vi "AlliGator Phasor Graph Context Menu Handler.vi"(8 "Error In":errorcluster, 9 "Help?":bool, 10 "Dialog? (T)":bool=TRUE, 11 "XY Graph Event":T3) -> (0 "Error Out":errorcluster, 1 "Message":string, 3 "AlliGator Actions":T1[](array[typedef]))   [LabVIEW 2021, in "AlliGator Phasor Graph.lvlib"]
doc: "Interprets Phasor Graph right-clic k menu items and sends corresponding actions to the action queue."
uses:
  AlliGator Phasor Graph.lvlib
  Graphs/XY Graph/XY Graph Event.ctl
  <vilib>/Utility/miscctls.llb/LVPoint32TypeDef.ctl
  AlliGator Q Element.ctl
  AlliGator Q Event.ctl
  Graphs/XY Graph/New Plot Information.ctl
  Graphs/Plot Scales.ctl
  Graphs/LabVIEW Plot Interpolation.ctl
  Graphs/Plot Point Style.ctl
  Graphs/XY Graph/XY Graph Selected Plot Info.ctl
  Graphs/XY Graph/XY Graph Refnum.ctl
  Graphs/XY Graph/XY Graph Mouse Click Event Data.ctl
  AlliGator Phasor Reference Data.ctl
  AlliGator Phasor Plot Scatter Plot Parameters.ctl
  AlliGator Phasor Graph Parameter List.ctl
  AlliGator Action Engine.lvlib
  Graphs/XY Graph/XY Graph Add-Ons.lvlib
  AlliGator Phasor Ratio.lvlib
  AlliGator Python Plugins.lvlib
  Graphs/Graphs.lvlib
panel:
  # "see the AlliGator License on the block diagram (Ctrl+E or Window:Show Block Diagram)"
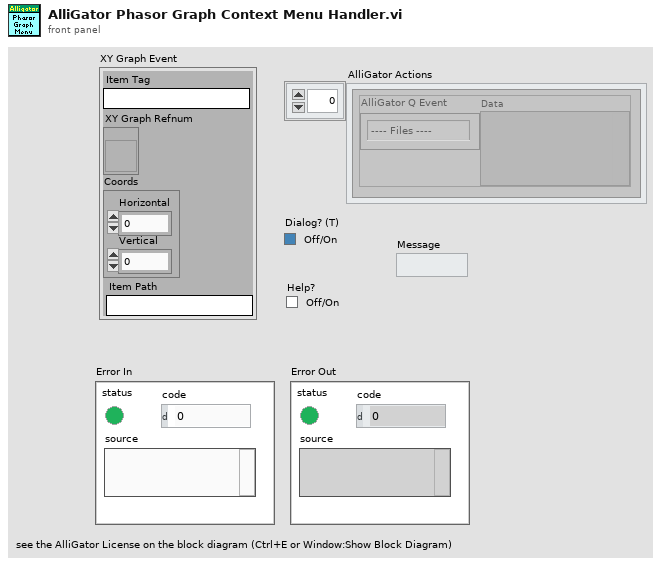
[diagram p1: front panel]
types:
  T1 = typedef "AlliGator Action Engine.lvlib/AlliGator Q Element.ctl" = cluster{"AlliGator Q Event":T2, "Data":variant}
  T2 = typedef "AlliGator Action Engine.lvlib/AlliGator Q Event.ctl" = enum16{"---- Files ----", "Files:Set Batch Export Files To Save", "Files:Set Dataset Loading & Pre-processing Options", "Files:Check #Frames in Dataset", "Files:Increment Frame Index", "Files:Open Mask Image", "Files:Open White Light Image", "Files:Open Single Dataset", "Files:New Folder of Folders Selected", "Files:Load File (all Types)_Scriptable", "Files:Move Flattened Series to Folders Series", "Files:Select Folder", "Files:Load FLI Dataset", "Files:Load Swiss SPAD 1 Dataset", "Files:Load Swiss SPAD 2 Dataset", "Files:Load .sdt FLI Dataset", "Files:Load .ptu FLI Dataset", "Files:Load .bin FLI Dataset", "Files:Load Single Gate Image Folder", "Files:Load I/m/phi Dataset (deprecated)", "Files:Load Single Image", "Files:Subtract Background File", "Files:Export FLI Dataset", "Files:Load HDF5 FLI Dataset", "Files:Set Destination File Path", "Files:Save Mask Image", "Files:Batch Conversion", "Files:New Folder Selected", "Files:Close FLI Dataset", "Files:Close FLI Dataset Series", "Files:Close White Light Image", "Files:Close Mask Image", "---- FLI Dataset ----", "FLI Dataset:Channel Arithmetic", "FLI Dataset:Export Average Lifetime Map as ASCII", "FLI Dataset:Export User-Defined Quantity Map as ASCII", "FLI Dataset:Python Function FLI Dataset Event", "FLI Dataset:ROI Analysis", "FLI Dataset:Tilted Logistic Square Gated IRF Characteristics Map", "FLI Dataset:Logistic Square Gated IRF Characteristics Map", "FLI Dataset:Square Gated IRF Characteristics Map", "FLI Dataset:Multi-ROI Single-Pixel Phasor Analysis", "FLI Dataset:Multi-ROI Single-Pixel NLSF Analysis", "FLI Dataset:All ROIs IRF Extraction", "FLI Dataset:All ROIs Decay Fit Non-Interactive (Fast + Individual IRF)", "FLI Dataset:All ROIs Phasor Analysis", "FLI Dataset:All ROIs Decay Fit", "FLI Dataset:Fluorescence Decay Statistics", "FLI Dataset:Update Decay Statistics Graph", "FLI Dataset:Get Decay from ROI", "FLI Dataset:All ROIs Average Lifetimes", "---- FLI Dataset Series ----", "FLI Dataset Series:Sum All Datasets in Series", "FLI Dataset Series:Add Dataset to Accumulated Dataset", "FLI Dataset Series:Display Accumulated Dataset", "FLI Dataset Series:Clear Dataset Series Sum", "FLI Dataset Series:Time-Series Analysis (NLSF)", "FLI Dataset Series:Time-Series Analysis (Phasor)", "---- Image ----", "Image:Update Image Profile Plots", "Image:Image Histogram Cursor Move", "Image:Image Histogram", "Image:Image Contrast", "Image:Set Image Histogram Cursor Move Flag", "Image:Clear Image Overlay", "Image:Use ROI as Search Area", "Image:Set ROI Diameter", "Image:Save Image Data as TIFF", "Image:Save Displayed Image with Overlay", "Image:Save Image Overlay Only", "Image:Save Image as Hot Pixel Mask", "Image:Change Source Image Color Palette", "Image:Copy Image to Clipboard", "Image:Source Image ROI Selection", "Image:Delete All ROIs", "Image:Delete All Unselected ROIs", "Image:Delete ROI", "Image:Merge All ROIs", "Image:Store ROI", "Image:Source Image ROI Storage", "Image:Export ROI Description to Notebook", "Image:Save ROI", "Image:Load ROI", "Image:Paste ROI Definition", "Image:Clear ROI", "Image:Identify ROIs in Mask Image", "Image:Create Complementary ROI", "Image:Create Contour ROI", "Image:Create ROI(s) from Pixels with Peak above Min_Scriptable", "Image:Create ROI(s) from Pixels with Intensity above Min_Scriptable", "Image:Compute ROI Statistics", "Image:Delete ROI(s) based on ROI Characteristics", "Image:Create ROI Grid", "Image:ROI to Individual Pixel ROIs", "Image:Python Function Source Image Event", "Image:Show Phasor Calibration Map ROI Centers", "Image:Convert ROI to Mask Image", "Image:Mouse Move", "Image:Mouse Up", "Image:Set Source Image Mouse Move Flag", "Image:Add Scale Bar Overlay", "Image:Delete Existing ROIs Option", "---- Decay ----", "Decay:Clear IRF/Reference Plot", "Decay:Clear Local IRFs", "Decay:Add Decay to Graph", "Decay:Smoothen Plot", "Decay:Smoothen Plot Tail", "Decay:Average Selected Plots", "Decay:Extract IRF", "Decay:Optimal IRF Extraction", "Decay:Threshold IRF", "Decay:Fit to Model IRF", "Decay:Fit IRF to Square Gate", "Decay:Fit IRF to Logistic Square Gate", "Decay:Fit IRF to Tilted Logistic Square Gate", "Decay:Create Bounding Cursors Set", "Decay:Export Bounding Cursors Definition to Notebook", "Decay:Denoise Plot", "Decay:Compute Cumulative Function", "Decay:Use as Reference Decay", "Decay:Show Reference Decay/IRF", "Decay:Extrapolate Decay", "Decay:Create Head & Tail Bounding Cursors", "Decay:Store Cursor-defined Head & Tail Fractions", "Decay:Rebin Plot", "Decay:1-Normalize Decay", "Decay:[0-1]-Normalize Plot", "Decay:Straighten Decay", "Decay:Shift Decay", "Decay:Fold Decay", "Decay:Fit Decay", "Decay:Global Fit of Selected Decays", "Decay:Post Global Fit Script", "Decay:Add Global Fit Parameters to Graph", "Decay:Add Decay Parameter(s) to Plot (Graph)", "Decay:Export Decay to Phasor Graph", "Decay:Plot Decay Shifts", "Decay:Compute Average Lifetime", "Decay:Plot Convolution", "Decay:Graph Tip Strip Update", "---- Decay Statistics ----", "Decay Statistics:Tip Strip Update", "---- Intensity Time Trace ----", "Intensity Time Trace:Use File Timestamp", "Intensity Time Trace:Load Intensity Corrections File", "Intensity Time Trace:Clear Intensity Corrections File", "Intensity Time Trace:Tip Strip Update", "---- Phasor Plot ----", "Phasor Plot:Build Phasor Plot", "Phasor Plot:Change Phasor Plot Color Palette", "Phasor Plot:Adjust Phasor Plot Display Range", "Phasor Plot:Highlight Image ROI in Phasor Plot", "Phasor Plot:Save Phasor Plot Image with Overlay", "Phasor Plot:Export Complex Phasor Map", "Phasor Plot:Export Phasor Ratio Map", "Phasor Plot:Export Average Lifetime Map", "Phasor Plot:Compute Phase Lifetime Histogram", "Phasor Plot:Compute Phasor Ratio Histogram", "Phasor Plot:Compute Phase Lifetime vs Intensity Scatter Plot", "Phasor Plot:Weber 2-Component Decomposition", "Phasor Plot:Update Phasor Color Map Vertices", "Phasor Plot:Clear Phasor Overlay", "Phasor Plot:Use Segment Extremities as References", "Phasor Plot:Use UC/Segment Intersections as References", "Phasor Plot:Use UC/Principal Axis Intersections as References", "Phasor Plot:Use UC/Linear Fit Intersections as References", "Phasor Plot:Update Phasor Plot Reference", "Phasor Plot:Show Local Phasor Info in Phasor Plot", "Phasor Plot:Update Phasor Plot State", "Phasor Plot:Phasor Plot ROI Storage", "Phasor Plot:Phasor Plot ROI Selection", "Phasor Plot:Python Function Phasor Plot Event", "Phasor Plot:Overlay Phasor ROI, Ratio or Map in Source Image", "Phasor Plot:Phasor at Image Pixel", "Phasor Plot:Mouse Move", "Phasor Plot:Mouse Up", "Phasor Plot:Display Range Mouse Move", "Phasor Plot:Set Mouse Move Flag", "---- Phasor Graph ----", "Phasor Graph:Calibrated Phasor Map Series", "Phasor Graph:Whole Image Phasor Scatter Plot (Todo)", "Phasor Graph:Get Phasor Value", "Phasor Graph:Create New Phasor Plot Dialog", "Phasor Graph:Update Last Phasor Value", "Phasor Graph:Update Phasor (m, phi)", "Phasor Graph:Remove Single Phasor from Plot", "Phasor Graph:Add Single Phasor to Plot", "Phasor Graph:Remove Phasor Plot", "Phasor Graph:Remove Selected Phasor Plots", "Phasor Graph:Clear Phasor Data", "Phasor Graph:Clear Phasor Graph", "Phasor Graph:Cursor Move", "Phasor Graph:Draw Cursor Connecting Line", "Phasor Graph:Clear Cursor Connecting Line", "Phasor Graph:Find UC Intersection", "Phasor Graph:Use UC/Cursor-Defined Line Intersections", "Phasor Graph:Use Selected Plots Fitted Line/UC Intersections", "Phasor Graph:Use Selected Plots Principal Axis/UC Intersections", "Phasor Graph:Show Single Phasor", "Phasor Graph:Save Single Phasor Plot", "Phasor Graph:Save All Phasor Plots", "Phasor Graph:Load Phasor Plot(s)", "Phasor Graph:Phasor Multiplication", "Phasor Graph:Compute Average Phasor", "Phasor Graph:Compute Multiple Average Phasors (Selected Plots)", "Phasor Graph:Export Single Phasor Plot Phase Lifetimes", "Phasor Graph:Phase Lifetime Trajectory", "Phasor Graph:Phase Lifetime vs Intensity Scatter Plot (deprecated)", "Phasor Graph:Parameter 2 vs Parameter 1 Scatter Plot", "Phasor Graph:Use Cursor n Location", "Phasor Graph:Set Reference n to Current Phase Lifetime Value", "Phasor Graph:Set Reference n to Lifetime Value", "Phasor Graph:Set Cursor n Location", "Phasor Graph:Save Phasor Graph Image", "Phasor Graph:Update SEPL Plot", "Phasor Graph:Export Single Phasor Plot Data", "Phasor Graph:Export Selected Phasor Plots Data", "Phasor Graph:Python Function Phasor Graph Event", "Phasor Graph:Tip Strip Update", "---- Calibration ----", "Calibration:Set Calibration Type", "Calibration:Load/Save Phasor Calibration", "Calibration:Load/Save Phasor Calibration Series", "Calibration:Load/Save Phasor Calibration Map", "Calibration:Use as Calibration", "Calibration:Compute Optimal Calibration from Phasor References", "Calibration:Clear Phasor Calibration", "Calibration:Use as Calibration Series", "Calibration:Use as Calibration Map", "Calibration:Clear Calibration Series", "Calibration:Clear Calibration Map", "Calibration:Apply Phasor Calibration", "Calibration:Update Single Plot Calibration", "Calibration:Update Multiple Plots Calibration", "Calibration:Clear Single Plot Calibration", "Calibration:Clear All Plots Calibrations", "Calibration:Clear Plot(s) Calibration(s)?", "Calibration:Phasor Calibration Maps (# Gates Series)", "---- Phasor Ratio ----", "Phasor Ratio:Clear Reference n", "Phasor Ratio:Toggle Selected Plot(s)  Lock to Reference 1", "Phasor Ratio:Use as Reference n", "Phasor Ratio:Send Reference n to Notebook", "Phasor Ratio:Toggle Selected Plot(s)  Lock to Reference 2", "Phasor Ratio:Compute Phasor Ratio at Mouse Location", "Phasor Ratio:Compute Phasor Plot's Average Phasor Ratio", "Phasor Ratio:Compute Time-Series Phasor Ratios", "Phasor Ratio:Fit Line to Phasor Ratio Plot", "Phasor Ratio:Save References", "Phasor Ratio:Load References", "Phasor Ratio:Update Phasor Reference 1", "Phasor Ratio:Update Phasor Reference 2", "Phasor Ratio:Move Cursor n to Reference n", "Phasor Ratio:Use as Phasor Reference 1 Lifetime", "Phasor Ratio:Use as Phasor Reference 2 Lifetime", "Phasor Ratio:Export Phasor Ratio Map as ASCII", "Phasor Ratio:Tip Strip Update", "---- Lifetime & Other Parameters Graph ----", "Lifetime:Tip Strip Update", "---- Decay Fit Parameter Map ----", "Decay Fit Parameter Map:Export ROI NLSF Data as ASCII", "Decay Fit Parameter Map:Set Decay Fit  Parameter Map Selection", "Decay Fit Parameter Map:Build Decay Fit Parameter Map", "Decay Fit Parameter Map:Change Decay Fit Parameter Map Color Palette", "Decay Fit Parameter Map:Export Decay Fit Parameter Map Data as ASCII", "Decay Fit Parameter Map:Export All Decay Fit Parameter Maps Data as ASCII", "Decay Fit Parameter Map:Send Map Data to Lifetime Graph", "Decay Fit Parameter Map:Save Decay Fit Parameter Map Image", "Decay Fit Parameter Map:Save-Load IRFs & Fit Data", "Decay Fit Parameter Map:Update Local Decay Plots", "Decay Fit Parameter Map:Python Function Decay Fit Parameters Map Event", "Decay Fit Parameter Map:Overlay Decay Fit Parameter Map in Source Image", "Decay Fit Parameter Map:Plot Map Data vs Intensity", "Decay Fit Parameter Map:Mouse Up", "Decay Fit Parameter Map:Display Range Mouse Move", "---- Generic Graph ----", "Generic Graph:Generic XY Graph Event", "Generic Graph:Python Function XY Graph Event", "Generic Graph:New Plot", "Generic Graph:Save Plot", "Generic Graph:XY Plot Histogram", "Generic Graph:Set XY Graph Plot Name", "Generic Graph:Set Last Cursor Style", "Generic Graph:Tip Strip Update", "---- GUI ----", "GUI:Start Script", "GUI:Type of Displayed Image Changed", "GUI:Gate Image Slide Changed", "GUI:Show Busy Icon", "GUI:Show Busy Icon & Abort Button", "GUI:Hide Busy Icon", "GUI:Hide Busy Icon & Abort Button", "GUI:Abort", "GUI:End Script", "GUI:Start Timing", "GUI:End Timing", "GUI:Set State Indicator", "GUI:Send Parameters JSON Strings to Clipboard", "GUI:Set Gate Step", "GUI:Idle", "GUI:Initialization", "GUI:Quit", "GUI:Increment Dataset Index", "GUI:Set Dataset Index to -1", "GUI:Time Series Slider Moved", "GUI:Time Series Slider Changed", "GUI:Toggle Playback or Loop", "GUI:Playback Script", "GUI:Set Phasor Frequency", "GUI:Open Window", "DEBUG"}
  T3 = typedef "XY Graph Add-Ons.lvlib/XY Graph Event.ctl" = cluster{"Item Tag":string, "XY Graph Refnum":refnum<vi>, "Coords":T4, "Item Path":string}
  T4 = typedef "LVPoint32TypeDef.ctl" = cluster{"Horizontal":i32, "Vertical":i32}
  T5 = typedef "XY Graph Add-Ons.lvlib/New Plot Information.ctl" = cluster{"Multiplot XY Graph":refnum<vi>, "Plot Name":string, "Plot Scales":T6, "Plot Interpolation":T7, "Point Style":T8, "Plot Color":u32, "Plot Metadata":variant}
  T6 = typedef "XY Graph Add-Ons.lvlib/Plot Scales.ctl" = cluster{"X Scale":u32, "Y Scale":u32}
  T7 = typedef "Graphs.lvlib/LabVIEW Plot Interpolation.ctl" = u8
  T8 = typedef "Graphs.lvlib/Plot Point Style.ctl" = enum16{"not defined", "None", "Empty Circle", "Filled Circle", "Thick Circle", "Dotted Circle", "Empty Square", "Filled Square", "Thick Square", "Dotted Square", "Small Filled Square", "Dot", "Cross", "Tiny Cross", "Large X", "Small x", "Diamond", "Small Empty Square"}
  T9 = typedef "XY Graph Add-Ons.lvlib/XY Graph Selected Plot Info.ctl" = cluster{"Multiplot XY Graph":T10, "Mouse Coordinates":T4, "Plot Index":i32}
  T10 = typedef "XY Graph Add-Ons.lvlib/XY Graph Refnum.ctl" = refnum<vi>
  T11 = typedef "XY Graph Add-Ons.lvlib/XY Graph Mouse Click Event Data.ctl" = cluster{"Multiplot XY Graph":T10, "Mouse Coordinates":T4}
  T12 = typedef "AlliGator Phasor Ratio.lvlib/AlliGator Phasor Reference Data.ctl" = cluster{"Data Type":string, "Data":variant}
  T13 = cluster{"Mouse Click Event Data":T11, "Save as...":bool}
  T14 = cluster{"XY Graph Refnum":refnum<vi>, "Coords":T4}
  T15 = cluster{cluster{"XY Graph Refnum":refnum<vi>, "Coords":T4}, i32}
  T16 = typedef "AlliGator Phasor Graph.lvlib/AlliGator Phasor Plot Scatter Plot Parameters.ctl" = cluster{"Parameter 2":T17, "Parameter 1":T17}
  T17 = typedef "AlliGator Phasor Graph.lvlib/AlliGator Phasor Graph Parameter List.ctl" = enum16{"Time Stamp", "Index", "Phasor Parameters", "Phasor g", "Phasor s", "Phasor phi", "Phasor m", "Modulus Lifetime", "Phase Lifetime", "ROI Parameters", "ROI Center x", "ROI Center y", "ROI # pixels ", "Decay Parameters", "Intensity", "Background/Gate", "Intensity - Background", "Fitted Lifetime", "Fitted Intensity", "Phasor Ratio Parameters", "Amplitude Phasor Ratio", "Intensity Phasor Ratio", "Amplitude-Averaged Lifetime", "Intensity-Averaged Lifetime", "-", "Phasor Parameters SDV", "Phasor g SDV", "Phasor s SDV", "Phasor phi SDV", "Phasor m SDV", "Phase Lifetime SDV", "Modulus Lifetime SDV", "Phasor Ratio Parameters SDV", "Amplitude Phasor Ratio SDV", "Intensity Phasor Ratio SDV", "Amplitude-Averaged Lifetime SDV", "Intensity-Averaged Lifetime SDV"}
  T18 = cluster{"Selected Plot Info":T9, "Dummy Scatter Plot Parameters\nindicating that a Dialog":T16}
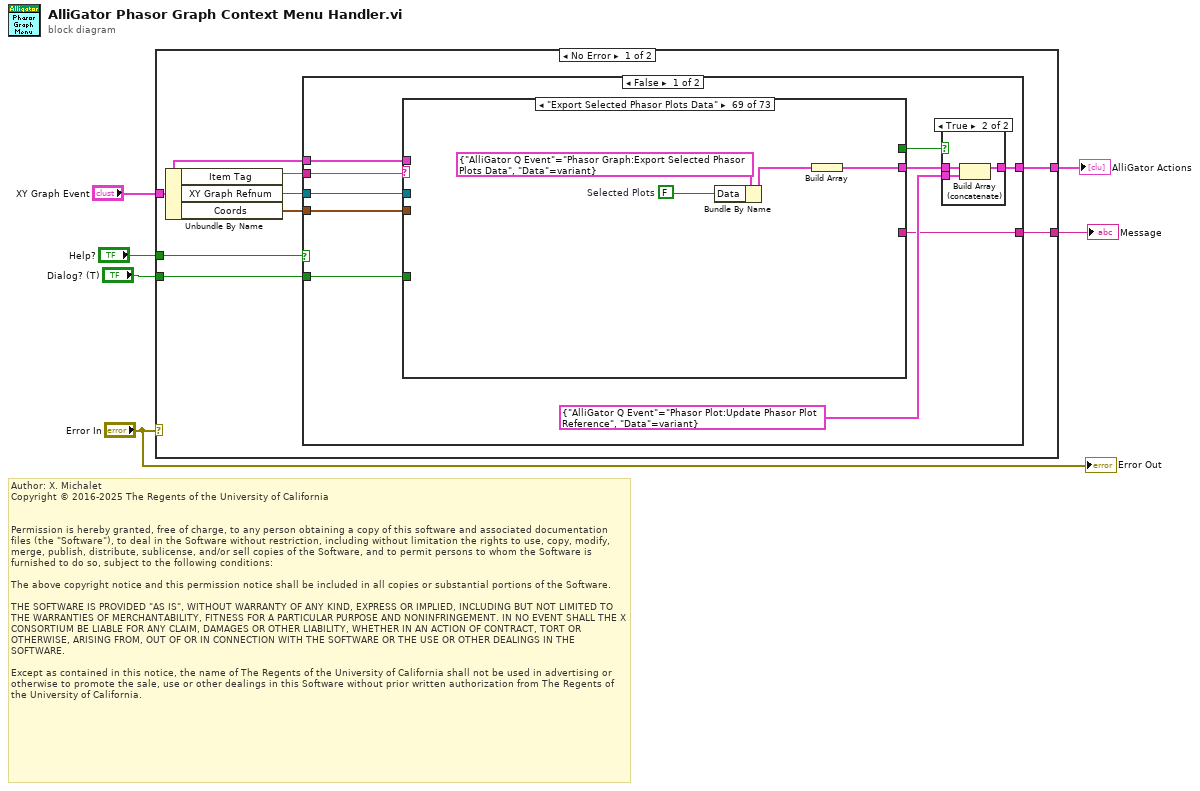
[diagram p0: block diagram]
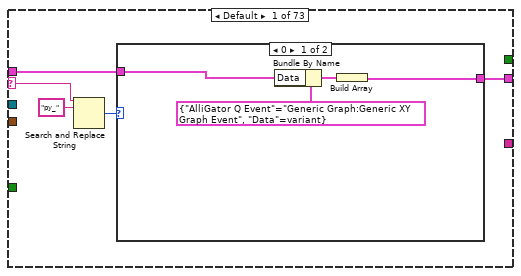
[diagram p3: hidden frame]
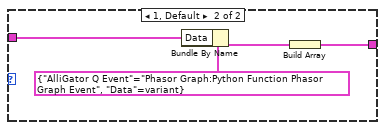
[diagram p4: hidden frame]
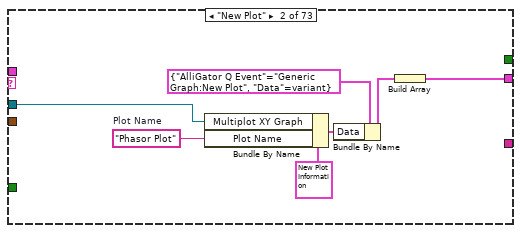
[diagram p5: hidden frame]
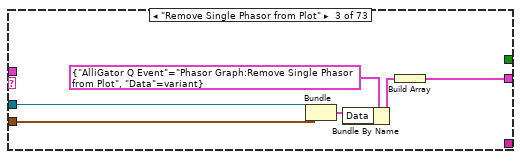
[diagram p6: hidden frame]
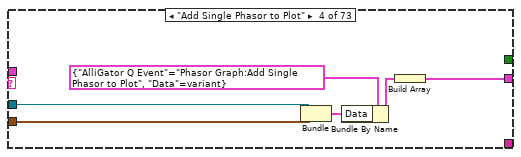
[diagram p7: hidden frame]
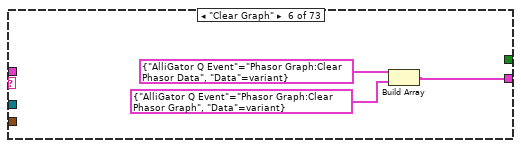
[diagram p9: hidden frame]
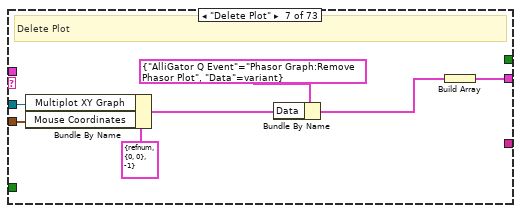
[diagram p10: hidden frame]
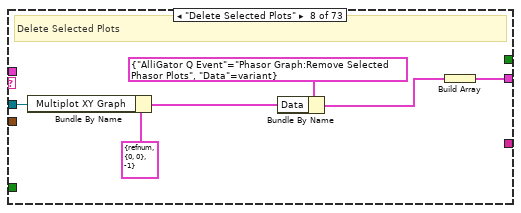
[diagram p11: hidden frame]
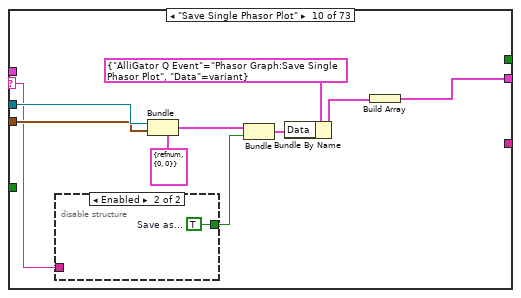
[diagram p13: hidden frame]
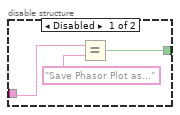
[diagram p14: hidden frame]
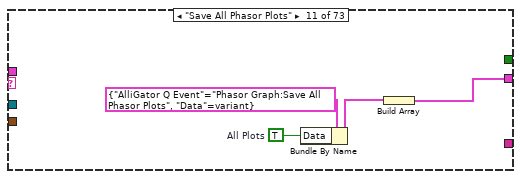
[diagram p15: hidden frame]
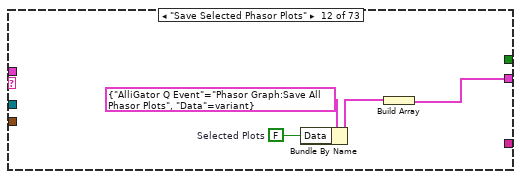
[diagram p16: hidden frame]
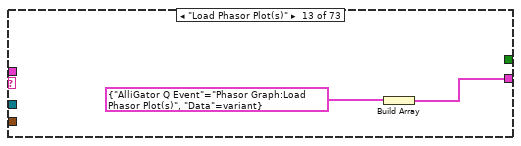
[diagram p17: hidden frame]
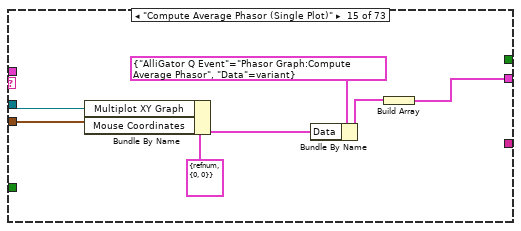
[diagram p19: hidden frame]
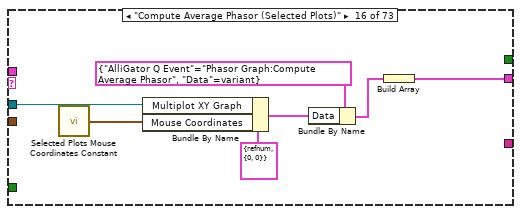
[diagram p20: hidden frame]
diagram:
  # "Author: X. Michalet\nCopyright © 2016-2025 The Regents of the University of California\n \n\nPermission is hereby granted, free of charge, to any person obtaining a copy of this software and associated documentation files (the \"Software\"), to deal in the Software without restriction, including without limitation the rights to use, copy, modify, merge, publish, distribute, sublicense, and/or sell copies of the Software, and to permit persons to whom the Software is furnished to do so, subject to the following conditions:\n\nThe above copyright notice and this permission notice shall be included in all copies or substantial portions of the Software.\n\nTHE SOFTWARE IS PROVIDED \"AS IS\", WITHOUT WARRANTY OF ANY KIND, EXPRESS OR IMPLIED, INCLUDING BUT NOT LIMITED TO THE WARRANTIES OF MERCHANTABILITY, FITNESS FOR A PARTICULAR PURPOSE AND NONINFRINGEMENT. IN NO EVENT SHALL THE X CONSORTIUM BE LIABLE FOR ANY CLAIM, DAMAGES OR OTHER LIABILITY, WHETHER IN AN ACTION OF CONTRACT, TORT OR OTHERWISE, ARISING FROM, OUT OF OR IN CONNECTION WITH THE SOFTWARE OR THE USE OR OTHER DEALINGS IN THE SOFTWARE.\n\nExcept as contained in this notice, the name of The Regents of the University of California shall not be used in advertising or otherwise to promote the sale, use or other dealings in this Software without prior written authorization from The Regents of the University of California."
  n1 = case shown="No Error" "Error In" {
    tunnel: [w11 _] -> w6
    tunnel: "XY Graph Event" -> [w10 _]
    tunnel: "Dialog? (T)" -> [w9 _]
    tunnel: "Help?" -> [w8 _]
    tunnel: [w7 _] -> w1
    frame No Error {
      n2 = Unbundle By Name(w10) -> ("Item Tag"=w14:string, "XY Graph Refnum"=w13:refnum<vi>, "Coords"=w12:T4)
      n3 = case shown="False" w8 {
        tunnel: w14 -> [w21 w382]
        tunnel: w13 -> [w20 w383]
        tunnel: w12 -> [w19 _]
        tunnel: [w18 _] -> w11
        tunnel: w10 -> [w17 _]
        tunnel: w9 -> [w16 _]
        tunnel: [w15 w381] -> w7
        frame False {
          n4 = case shown="\"Export Selected Phasor Plots Data\"" w21 {
            selector: w21 -> [w29 _ _ _ _ _ _ _ _ w79 _ _ _ _ _ _ _ _ _ _ _ _ _ _ _ _ _ _ _ _ _ _ _ _ _ _ _ _ w190 w204 _ _ _ _ _ w268 _ w283 _ _ _ _ _ _ _ _ _ _ _ _ _ _ _ _ _ _ _ _ _ _ _ _ _]
            tunnel: w20 -> [_ w48 w54 w60 _ _ w70 w76 _ w84 _ _ _ _ w103 w111 w118 _ _ _ _ _ _ w129 _ _ w136 _ _ w143 w150 _ _ _ _ _ _ _ w194 _ _ _ w231 _ _ _ _ _ _ _ _ _ _ _ _ _ w313 w319 w323 _ w329 _ w338 w347 w356 _ _ w368 _ _ _ w378 w380]
            tunnel: w19 -> [_ _ w53 w59 _ _ w69 _ _ w83 _ _ _ _ w104 _ _ _ _ _ _ _ _ w128 _ _ w135 _ _ w144 w151 _ _ _ _ _ _ _ w193 _ _ _ _ _ _ _ _ _ _ _ _ _ _ _ _ _ w312 w318 w322 _ w328 _ w337 _ _ _ _ w367 _ _ _ _ _]
            tunnel: [w33 w43 w49 w55 _ w61 w65 w72 _ w77 w91 w95 w99 _ w101 w109 w116 T1[] [{"AlliGator Q Event"=enum."Phasor Graph:Phasor Multiplication", "Data"=variant}] ("element") _ T1[] [{"AlliGator Q Event"=enum."Calibration:Use as Calibration", "Data"=variant}] ("element") T1[] [{"AlliGator Q Event"=enum."Calibration:Compute Optimal Calibration from Phasor References", "Data"=variant}] ("element") T1[] [{"AlliGator Q Event"=enum."Calibration:Clear Phasor Calibration", "Data"=variant}] ("element") _ w126 T1[] [{"AlliGator Q Event"=enum."Calibration:Clear Calibration Series", "Data"=variant}] ("element") _ w133 T1[] [{"AlliGator Q Event"=enum."Calibration:Clear Calibration Map", "Data"=variant}] ("element") _ w140 w147 w154 w158 w162 w166 _ w171 w176 w186 w201 w210 w229 w239 w250 w261 w265 w272 w279 w286 T1[] [{"AlliGator Q Event"=enum."Phasor Ratio:Save References", "Data"=variant}] ("element") T1[] [{"AlliGator Q Event"=enum."Phasor Ratio:Load References", "Data"=variant}] ("element") w297 w301 w303 w305 _ w308 w314 w320 _ w326 _ w336 w346 w355 w359 _ w365 w372 w376 _ _ _] -> w22
            tunnel: [_ _ _ _ _ _ _ _ _ _ _ _ _ _ _ _ _ _ _ _ _ _ _ _ _ _ _ _ _ _ _ _ _ _ _ _ TRUE TRUE TRUE TRUE TRUE TRUE TRUE TRUE TRUE TRUE TRUE TRUE TRUE _ TRUE _ _ _ _ _ _ _ _ _ _ _ _ _ _ _ _ _ _ _ _ _ _] -> w24
            tunnel: w16 -> [_ _ _ _ _ _ _ _ _ _ _ _ _ _ _ _ _ _ _ _ _ _ _ _ _ _ _ _ _ _ _ _ _ _ _ _ _ _ _ _ _ _ _ _ _ _ _ _ _ _ _ _ _ _ _ _ _ _ _ _ _ _ _ _ _ _ _ w366 _ _ _ _ _]
            tunnel: w17 -> [w30 _ _ _ _ _ _ _ _ _ _ _ _ _ _ _ _ _ _ _ _ _ _ _ _ _ _ _ _ _ _ _ _ _ _ _ _ _ _ _ _ _ _ _ _ _ _ _ _ _ _ _ _ _ _ _ _ _ _ _ _ _ _ _ _ _ _ _ _ _ _ _ _]
            tunnel: [_ _ _ _ _ _ _ _ _ _ _ _ _ _ _ _ _ _ _ _ _ _ _ _ _ _ _ _ _ _ _ _ _ _ _ _ _ _ _ _ _ _ _ _ _ _ _ _ _ _ _ _ _ _ _ _ _ _ _ _ _ _ _ _ _ _ _ _ _ _ _ w377 w379] -> w15
            frame Default {
              n5 = Search and Replace String(input string=w29, search string="py_") -> (number of replacements=w31:i32)  [unwired: 6 in, 3 out]
              n6 = case shown="0" w31 {
                tunnel: [w34 w39] -> w33
                tunnel: w30 -> [w35 w38]
                frame 0 {
                  n7 = Bundle By Name(cluster=T1 {"AlliGator Q Event"=enum."Generic Graph:Generic XY Graph Event", "Data"=variant} ("element"), "Data"=w35) -> (w37:T1)
                  n8 = Build Array(w37) -> (w34:T1[])
                }
                frame 1, Default {
                  n9 = Bundle By Name(cluster=T1 {"AlliGator Q Event"=enum."Phasor Graph:Python Function Phasor Graph Event", "Data"=variant}, "Data"=w38) -> (w40:T1)
                  n10 = Build Array(w40) -> (w39:T1[])
                }
              }
            }
            frame "New Plot" {
              w45 = "Phasor Plot"  # Plot Name
              n11 = Bundle By Name(cluster=T5 {"Multiplot XY Graph"=refnum, "Plot Name"="", "Plot Scales"={"X Scale"=0, "Y Scale"=0}, "Plot Interpolation"=0, "Point Style"=enum."Empty Square", "Plot Color"=15781887, "Plot Metadata"=variant} ("New Plot Information"), "Multiplot XY Graph"=w48, "Plot Name"=w45) -> (w46:T5)
              n12 = Bundle By Name(cluster=T1 {"AlliGator Q Event"=enum."Generic Graph:New Plot", "Data"=variant} ("element"), "Data"=w46) -> (w47:T1)
              n13 = Build Array(w47) -> (w43:T1[])
            }
            frame "Remove Single Phasor from Plot" {
              n14 = Bundle("XY Graph Refnum"=w54, "Coords"=w53) -> (w50:T14)  [unwired: 1 in]
              n15 = Bundle By Name(cluster=T1 {"AlliGator Q Event"=enum."Phasor Graph:Remove Single Phasor from Plot", "Data"=variant} ("element"), "Data"=w50) -> (w51:T1)
              n16 = Build Array(w51) -> (w49:T1[])
            }
            frame "Add Single Phasor to Plot" {
              n17 = Bundle("XY Graph Refnum"=w60, "Coords"=w59) -> (w56:T14)  [unwired: 1 in]
              n18 = Bundle By Name(cluster=T1 {"AlliGator Q Event"=enum."Phasor Graph:Add Single Phasor to Plot", "Data"=variant} ("element"), "Data"=w56) -> (w57:T1)
              n19 = Build Array(w57) -> (w55:T1[])
            }
            frame "------------------------" {
            }
            frame "Clear Graph" {
              n20 = Build Array(T1 {"AlliGator Q Event"=enum."Phasor Graph:Clear Phasor Data", "Data"=variant} ("element"), T1 {"AlliGator Q Event"=enum."Phasor Graph:Clear Phasor Graph", "Data"=variant} ("element")) -> (w61:T1[])
            }
            frame "Delete Plot" {
              # "Delete Plot"
              n21 = Bundle By Name(cluster=T9 {"Multiplot XY Graph"=refnum, "Mouse Coordinates"={"Horizontal"=0, "Vertical"=0}, "Plot Index"=-1} ("Selected Plot Info"), "Multiplot XY Graph"=w70, "Mouse Coordinates"=w69) -> (w68:T9)
              n22 = Bundle By Name(cluster=T1 {"AlliGator Q Event"=enum."Phasor Graph:Remove Phasor Plot", "Data"=variant} ("element"), "Data"=w68) -> (w66:T1)
              n23 = Build Array(w66) -> (w65:T1[])
            }
            frame "Delete Selected Plots" {
              # "Delete Selected Plots"
              n24 = Bundle By Name(cluster=T9 {"Multiplot XY Graph"=refnum, "Mouse Coordinates"={"Horizontal"=0, "Vertical"=0}, "Plot Index"=-1} ("Selected Plot Info"), "Multiplot XY Graph"=w76) -> (w75:T9)
              n25 = Bundle By Name(cluster=T1 {"AlliGator Q Event"=enum."Phasor Graph:Remove Selected Phasor Plots", "Data"=variant} ("element"), "Data"=w75) -> (w73:T1)
              n26 = Build Array(w73) -> (w72:T1[])
            }
            frame "---------------------------" {
            }
            frame "Save Single Phasor Plot" {
              n27 = disable-structure shown="Enabled" {
                disable-tunnel: w79 -> [w89 _]
                disable-tunnel: [w87 w90] -> w78
                frame Disabled {
                  n28 = Equal?(x=w89, y="Save Phasor Plot as...") -> (x = y?=w87:bool)
                }
                frame Enabled {
                  w90 = TRUE  # Save as...
                }
              }
              n29 = Bundle(cluster=T11 {"Multiplot XY Graph"=refnum, "Mouse Coordinates"={"Horizontal"=0, "Vertical"=0}} ("Mouse Click Event Data"), "Multiplot XY Graph"=w84, "Mouse Coordinates"=w83) -> (w81:T11)
              n30 = Bundle("Mouse Click Event Data"=w81, "Save as..."=w78) -> (w80:T13)  [unwired: 1 in]
              n31 = Bundle By Name(cluster=T1 {"AlliGator Q Event"=enum."Phasor Graph:Save Single Phasor Plot", "Data"=variant} ("element"), "Data"=w80) -> (w85:T1)
              n32 = Build Array(w85) -> (w77:T1[])
            }
            frame "Save All Phasor Plots" {
              w92 = TRUE  # All Plots
              n33 = Bundle By Name(cluster=T1 {"AlliGator Q Event"=enum."Phasor Graph:Save All Phasor Plots", "Data"=variant} ("element"), "Data"=w92) -> (w93:T1)
              n34 = Build Array(w93) -> (w91:T1[])
            }
            frame "Save Selected Phasor Plots" {
              w96 = FALSE  # Selected Plots
              n35 = Bundle By Name(cluster=T1 {"AlliGator Q Event"=enum."Phasor Graph:Save All Phasor Plots", "Data"=variant} ("element"), "Data"=w96) -> (w97:T1)
              n36 = Build Array(w97) -> (w95:T1[])
            }
            frame "Load Phasor Plot(s)" {
              n37 = Build Array(T1 {"AlliGator Q Event"=enum."Phasor Graph:Load Phasor Plot(s)", "Data"=variant} ("element")) -> (w99:T1[])
            }
            frame "-------Phasor Math----------" {
            }
            frame "Compute Average Phasor (Single Plot)" {
              n38 = Bundle By Name(cluster=T11 {"Multiplot XY Graph"=refnum, "Mouse Coordinates"={"Horizontal"=0, "Vertical"=0}} ("Mouse Click Event Data"), "Multiplot XY Graph"=w103, "Mouse Coordinates"=w104) -> (w102:T11)
              n39 = Bundle By Name(cluster=T1 {"AlliGator Q Event"=enum."Phasor Graph:Compute Average Phasor", "Data"=variant} ("element"), "Data"=w102) -> (w106:T1)
              n40 = Build Array(w106) -> (w101:T1[])
            }
            frame "Compute Average Phasor (Selected Plots)" {
              n41 = call "Selected Plots Mouse Coordinates Constant.vi"() -> ("Selected Plots Mouse Coordinates Equivalent"=w108:T4)
              n42 = Bundle By Name(cluster=T11 {"Multiplot XY Graph"=refnum, "Mouse Coordinates"={"Horizontal"=0, "Vertical"=0}} ("Mouse Click Event Data"), "Multiplot XY Graph"=w111, "Mouse Coordinates"=w108) -> (w110:T11)
              n43 = Bundle By Name(cluster=T1 {"AlliGator Q Event"=enum."Phasor Graph:Compute Average Phasor", "Data"=variant} ("element"), "Data"=w110) -> (w113:T1)
              n44 = Build Array(w113) -> (w109:T1[])
            }
            frame "Compute Average Phasor (All Plots)" {
              n45 = call "All Plots Mouse Coordinates Constant.vi"() -> ("Selected Plots Mouse Coordinates Equivalent"=w115:T4)
              n46 = Bundle By Name(cluster=T11 {"Multiplot XY Graph"=refnum, "Mouse Coordinates"={"Horizontal"=0, "Vertical"=0}} ("Mouse Click Event Data"), "Multiplot XY Graph"=w118, "Mouse Coordinates"=w115) -> (w117:T11)
              n47 = Bundle By Name(cluster=T1 {"AlliGator Q Event"=enum."Phasor Graph:Compute Average Phasor", "Data"=variant} ("element"), "Data"=w117) -> (w120:T1)
              n48 = Build Array(w120) -> (w116:T1[])
            }
            frame "Phasor Multiplication" {
            }
            frame "---- Phasor Calibration Definition ----" {
            }
            frame "Use Current Phasor as Calibration" {
            }
            frame "Compute Optimal Calibration from Phasor References" {
            }
            frame "Clear Single Phasor Calibration" {
            }
            frame "---- Time-Series Calibration Definition ----" {
            }
            frame "Use as Phasor Calibration Series" {
              n49 = Bundle("XY Graph Refnum"=w129, "Coords"=w128) -> (w127:T14)  [unwired: 1 in]
              n50 = Bundle By Name(cluster=T1 {"AlliGator Q Event"=enum."Calibration:Use as Calibration Series", "Data"=variant} ("element"), "Data"=w127) -> (w130:T1)
              n51 = Build Array(w130) -> (w126:T1[])
            }
            frame "Clear Phasor Calibration Series" {
            }
            frame "-------- Phasor Calibration Map -----------" {
            }
            frame "Use as Phasor Calibration Map" {
              n52 = Bundle("XY Graph Refnum"=w136, "Coords"=w135) -> (w134:T14)  [unwired: 1 in]
              n53 = Bundle By Name(cluster=T1 {"AlliGator Q Event"=enum."Calibration:Use as Calibration Map", "Data"=variant} ("element"), "Data"=w134) -> (w137:T1)
              n54 = Build Array(w137) -> (w133:T1[])
            }
            frame "Clear Phasor Calibration Map" {
            }
            frame "-----------------------------------" {
            }
            frame "Update Single Plot Calibration" {
              n55 = Bundle(cluster=T11 {"Multiplot XY Graph"=refnum, "Mouse Coordinates"={"Horizontal"=0, "Vertical"=0}} ("Mouse Click Event Data"), "Multiplot XY Graph"=w143, "Mouse Coordinates"=w144) -> (w142:T11)
              n56 = Bundle By Name(cluster=T1 {"AlliGator Q Event"=enum."Calibration:Update Single Plot Calibration", "Data"=variant} ("element"), "Data"=w142) -> (w145:T1)
              n57 = Build Array(w145) -> (w140:T1[])
            }
            frame "Clear Single Plot Calibration" {
              n58 = Bundle(cluster=T11 {"Multiplot XY Graph"=refnum, "Mouse Coordinates"={"Horizontal"=0, "Vertical"=0}} ("Mouse Click Event Data"), "Multiplot XY Graph"=w150, "Mouse Coordinates"=w151) -> (w149:T11)
              n59 = Bundle By Name(cluster=T1 {"AlliGator Q Event"=enum."Calibration:Clear Single Plot Calibration", "Data"=variant} ("element"), "Data"=w149) -> (w152:T1)
              n60 = Build Array(w152) -> (w147:T1[])
            }
            frame "Update All Plots Calibrations" {
              n61 = Bundle By Name(cluster=T1 {"AlliGator Q Event"=enum."Calibration:Update Multiple Plots Calibration", "Data"=variant} ("element"), "Data"=TRUE) -> (w156:T1)
              n62 = Build Array(w156) -> (w154:T1[])
            }
            frame "Update Selected Plots Calibrations" {
              n63 = Bundle By Name(cluster=T1 {"AlliGator Q Event"=enum."Calibration:Update Multiple Plots Calibration", "Data"=variant} ("element"), "Data"=FALSE) -> (w160:T1)
              n64 = Build Array(w160) -> (w158:T1[])
            }
            frame "Clear All Plots Calibrations" {
              w163 = TRUE  # All Plots
              n65 = Bundle By Name(cluster=T1 {"AlliGator Q Event"=enum."Calibration:Clear All Plots Calibrations", "Data"=variant} ("Time-Gated Phasor Q Element"), "Data"=w163) -> (w165:T1)
              n66 = Build Array(w165) -> (w162:T1[])
            }
            frame "Clear Selected Plots Calibrations" {
              w167 = FALSE  # Selected Plots
              n67 = Bundle By Name(cluster=T1 {"AlliGator Q Event"=enum."Calibration:Clear All Plots Calibrations", "Data"=variant} ("Time-Gated Phasor Q Element"), "Data"=w167) -> (w169:T1)
              n68 = Build Array(w169) -> (w166:T1[])
            }
            frame "---- Phasor Ratio Reference ----" {
            }
            frame "Set Reference 1 to User-entered Lifetime" {
              n69 = Bundle By Name(cluster=T1 {"AlliGator Q Event"=enum."Phasor Graph:Set Reference n to Lifetime Value", "Data"=variant} ("element"), "Data"=1) -> (w173:T1)
              n70 = Build Array(w173) -> (w171:T1[])
            }
            frame "Set Reference 2 to User-entered Lifetime" {
              n71 = Bundle By Name(cluster=T1 {"AlliGator Q Event"=enum."Phasor Graph:Set Reference n to Lifetime Value", "Data"=variant} ("element"), "Data"=2) -> (w178:T1)
              n72 = Build Array(w178) -> (w176:T1[])
            }
            frame "Use as Reference 1", "Use as Reference 2" {
              n73 = Bundle("XY Graph Refnum"=w194, "Coords"=w193) -> (w188:T14)  [unwired: 1 in]
              n74 = Scan From String(format string="Use as Reference %d", input string=w190) -> (output 1=w184:i32)  [unwired: 3 in, 3 out]
              n75 = Bundle(w188, w184) -> (w182:T15)  [unwired: 1 in]
              n76 = Bundle By Name(cluster=T12 {"Data Type"="Phasor Graph", "Data"=variant} ("Phasor Reference Data"), "Data"=w182) -> (w181:T12)
              n77 = Bundle By Name(cluster=T1 {"AlliGator Q Event"=enum."Phasor Ratio:Use as Reference n", "Data"=variant} ("element"), "Data"=w181) -> (w191:T1)
              n78 = Bundle By Name(cluster=T1 {"AlliGator Q Event"=enum."Phasor Ratio:Send Reference n to Notebook", "Data"=variant} ("element"), "Data"=w184) -> (w183:T1)
              n79 = Build Array(w191, w183) -> (w186:T1[])
            }
            frame "Use Cursor 1 as Reference 1", "Use Cursor 2 as Reference 2" {
              n80 = Scan From String(format string="Use Cursor %d as Reference %d", input string=w204) -> (output 1=w197:i32)  [unwired: 5 in, 3 out]
              n81 = Bundle By Name(cluster=T12 {"Data Type"="Last Phasor", "Data"=variant} ("Phasor Reference Data"), "Data"=w197) -> (w196:T12)
              n82 = Bundle By Name(cluster=T1 {"AlliGator Q Event"=enum."Phasor Ratio:Send Reference n to Notebook", "Data"=variant} ("element"), "Data"=w197) -> (w198:T1)
              n83 = Bundle By Name(cluster=T1 {"AlliGator Q Event"=enum."Phasor Graph:Use Cursor n Location", "Data"=variant} ("element"), "Data"=w197) -> (w206:T1)
              n84 = Bundle By Name(cluster=T1 {"AlliGator Q Event"=enum."Phasor Ratio:Use as Reference n", "Data"=variant} ("element"), "Data"=w196) -> (w202:T1)
              n85 = Build Array(w206, w202, w198) -> (w201:T1[])
            }
            frame "Use Cursors 1 & 2 as References 1 & 2" {
              n86 = for {
                N: 2 -> [_]
                tunnel: [w220] -> w210 mode=concatenating
                i -> [w216]
                n87 = Increment(x=w216) -> (x+1=w212:i32)
                n88 = Bundle By Name(cluster=T12 {"Data Type"="Last Phasor", "Data"=variant} ("Phasor Reference Data"), "Data"=w212) -> (w211:T12)
                n89 = Bundle By Name(cluster=T1 {"AlliGator Q Event"=enum."Phasor Graph:Use Cursor n Location", "Data"=variant} ("element"), "Data"=w212) -> (w219:T1)
                n90 = Bundle By Name(cluster=T1 {"AlliGator Q Event"=enum."Phasor Ratio:Send Reference n to Notebook", "Data"=variant} ("element"), "Data"=w212) -> (w214:T1)
                n91 = Bundle By Name(cluster=T1 {"AlliGator Q Event"=enum."Phasor Ratio:Use as Reference n", "Data"=variant} ("element"), "Data"=w211) -> (w217:T1)
                n92 = Build Array(w219, w217, w214) -> (w220:T1[])
              }
            }
            frame "Use UC/Cursor-Defined Line Intersections" {
              n93 = Bundle By Name(cluster=T1 {"AlliGator Q Event"=enum."Phasor Ratio:Send Reference n to Notebook", "Data"=variant} ("element"), "Data"=2) -> (w224:T1)
              n94 = Bundle By Name(cluster=T1 {"AlliGator Q Event"=enum."Phasor Ratio:Send Reference n to Notebook", "Data"=variant} ("element"), "Data"=1) -> (w225:T1)
              n95 = Build Array(T1 {"AlliGator Q Event"=enum."Phasor Graph:Use UC/Cursor-Defined Line Intersections", "Data"=variant} ("element"), w225, w224) -> (w229:T1[])
            }
            frame "Use Selected Plots Fitted Line/UC Intersections" {
              n96 = Bundle By Name(cluster=T1 {"AlliGator Q Event"=enum."Phasor Ratio:Send Reference n to Notebook", "Data"=variant} ("element"), "Data"=2) -> (w232:T1)
              n97 = Bundle By Name(cluster=T1 {"AlliGator Q Event"=enum."Phasor Ratio:Send Reference n to Notebook", "Data"=variant} ("element"), "Data"=1) -> (w233:T1)
              n98 = Bundle By Name(cluster=T1 {"AlliGator Q Event"=enum."Phasor Graph:Use Selected Plots Fitted Line/UC Intersections", "Data"=variant} ("element"), "Data"=w231) -> (w240:T1)
              n99 = Build Array(w240, w233, w232) -> (w239:T1[])
            }
            frame "Use Selected Plots Major Axis/UC Intersections" {
              n100 = Bundle By Name(cluster=T1 {"AlliGator Q Event"=enum."Phasor Ratio:Send Reference n to Notebook", "Data"=variant} ("element"), "Data"=2) -> (w243:T1)
              n101 = Bundle By Name(cluster=T1 {"AlliGator Q Event"=enum."Phasor Ratio:Send Reference n to Notebook", "Data"=variant} ("element"), "Data"=1) -> (w244:T1)
              n102 = Bundle By Name(cluster=T1 {"AlliGator Q Event"=enum."Phasor Graph:Use Selected Plots Principal Axis/UC Intersections", "Data"=variant} ("element"), "Data"=TRUE) -> (w251:T1)
              n103 = Build Array(w251, w244, w243) -> (w250:T1[])
            }
            frame "Use Selected Plots Minor Axis/UC Intersections" {
              n104 = Bundle By Name(cluster=T1 {"AlliGator Q Event"=enum."Phasor Ratio:Send Reference n to Notebook", "Data"=variant} ("element"), "Data"=2) -> (w254:T1)
              n105 = Bundle By Name(cluster=T1 {"AlliGator Q Event"=enum."Phasor Ratio:Send Reference n to Notebook", "Data"=variant} ("element"), "Data"=1) -> (w255:T1)
              n106 = Bundle By Name(cluster=T1 {"AlliGator Q Event"=enum."Phasor Graph:Use Selected Plots Principal Axis/UC Intersections", "Data"=variant} ("element"), "Data"=FALSE) -> (w262:T1)
              n107 = Build Array(w262, w255, w254) -> (w261:T1[])
            }
            frame "Move Cursor 1 to Reference 1", "Move Cursor 2 to Reference 2" {
              n108 = Scan From String(format string="Move Cursor %d to Reference %d", input string=w268) -> (output 1=w266:i32)  [unwired: 5 in, 3 out]
              n109 = Bundle By Name(cluster=T1 {"AlliGator Q Event"=enum."Phasor Ratio:Move Cursor n to Reference n", "Data"=variant} ("element"), "Data"=w266) -> (w269:T1)
              n110 = Build Array(w269) -> (w265:T1[])
            }
            frame "Move Cursors 1 & 2 to References 1 & 2" {
              n111 = for {
                N: 2 -> [_]
                tunnel: [w276] -> w272 mode=indexing
                i -> [w275]
                n112 = Increment(x=w275) -> (x+1=w274:i32)
                n113 = Bundle By Name(cluster=T1 {"AlliGator Q Event"=enum."Phasor Ratio:Move Cursor n to Reference n", "Data"=variant} ("element"), "Data"=w274) -> (w276:T1)
              }
            }
            frame "Clear Reference 1", "Clear Reference 2" {
              n114 = Scan From String(format string="Clear Reference %d", input string=w283) -> (output 1=w281:i32)  [unwired: 3 in, 3 out]
              n115 = Bundle By Name(cluster=T1 {"AlliGator Q Event"=enum."Phasor Ratio:Clear Reference n", "Data"=variant} ("Time-Gated Phasor Q Element"), "Data"=w281) -> (w280:T1)
              n116 = Build Array(w280) -> (w279:T1[])
            }
            frame "Clear All References" {
              w290 = T1 {"AlliGator Q Event"=enum."Phasor Ratio:Clear Reference n", "Data"=variant} ("Time-Gated Phasor Q Element")
              n117 = Bundle By Name(cluster=w290, "Data"=1) -> (w288:T1)
              n118 = Bundle By Name(cluster=w290, "Data"=2) -> (w287:T1)
              n119 = Build Array(w288, w287) -> (w286:T1[])
            }
            frame "Save References" {
            }
            frame "Load References" {
            }
            frame "Export Reference 1 to Notebook" {
              n120 = Bundle By Name(cluster=T1 {"AlliGator Q Event"=enum."Phasor Ratio:Send Reference n to Notebook", "Data"=variant} ("element"), "Data"=1) -> (w296:T1)
              n121 = Build Array(w296) -> (w297:T1[])
            }
            frame "Export Reference 2 to Notebook" {
              n122 = Bundle By Name(cluster=T1 {"AlliGator Q Event"=enum."Phasor Ratio:Send Reference n to Notebook", "Data"=variant} ("element"), "Data"=2) -> (w300:T1)
              n123 = Build Array(w300) -> (w301:T1[])
            }
            frame "Toggle Selected Plot(s) to Lock to Reference 1" {
              n124 = Build Array(T1 {"AlliGator Q Event"=enum."Phasor Ratio:Toggle Selected Plot(s)  Lock to Reference 1", "Data"=variant} ("element")) -> (w303:T1[])
            }
            frame "Toggle Selected Plot(s) to Lock to Reference 2" {
              n125 = Build Array(T1 {"AlliGator Q Event"=enum."Phasor Ratio:Toggle Selected Plot(s)  Lock to Reference 2", "Data"=variant} ("element")) -> (w305:T1[])
            }
            frame "---- Phasor Ratio Calculation ----" {
            }
            frame "Compute Single Phasor Ratio at Mouse Location" {
              n126 = Bundle(cluster=T11 {"Multiplot XY Graph"=refnum, "Mouse Coordinates"={"Horizontal"=0, "Vertical"=0}} ("Mouse Click Event Data"), "Multiplot XY Graph"=w313, "Mouse Coordinates"=w312) -> (w309:T11)
              n127 = Bundle By Name(cluster=T1 {"AlliGator Q Event"=enum."Phasor Ratio:Compute Phasor Ratio at Mouse Location", "Data"=variant} ("element"), "Data"=w309) -> (w310:T1)
              n128 = Build Array(w310) -> (w308:T1[])
            }
            frame "Compute Phasor Plot's Average Phasor Ratio" {
              n129 = Bundle("XY Graph Refnum"=w319, "Coords"=w318) -> (w315:T14)  [unwired: 1 in]
              n130 = Bundle By Name(cluster=T1 {"AlliGator Q Event"=enum."Phasor Ratio:Compute Phasor Plot's Average Phasor Ratio", "Data"=variant} ("element"), "Data"=w315) -> (w316:T1)
              n131 = Build Array(w316) -> (w314:T1[])
            }
            frame "Compute Time-Series Phasor Ratios" {
              n132 = Bundle("XY Graph Refnum"=w323, "Coords"=w322) -> (w321:T14)  [unwired: 1 in]
              n133 = Bundle By Name(cluster=T1 {"AlliGator Q Event"=enum."Phasor Ratio:Compute Time-Series Phasor Ratios", "Data"=variant} ("element"), "Data"=w321) -> (w324:T1)
              n134 = Build Array(w324) -> (w320:T1[])
            }
            frame "-------------------------" {
            }
            frame "Phase Lifetime Series" {
              n135 = Bundle("XY Graph Refnum"=w329, "Coords"=w328) -> (w327:T14)  [unwired: 1 in]
              n136 = Bundle By Name(cluster=T1 {"AlliGator Q Event"=enum."Phasor Graph:Phase Lifetime Trajectory", "Data"=variant} ("element"), "Data"=w327) -> (w330:T1)
              n137 = Build Array(w330) -> (w326:T1[])
            }
            frame "---- Parameter 2 vs Parameter 1 Scatter Plot ----" {
            }
            frame "Parameter 2 vs Parameter 1 Scatter Plot (Single Plot)" {
              w335 = T16 {"Parameter 2"=enum."Phasor g", "Parameter 1"=enum."Phasor g"}  # Dummy Scatter Plot Parameters indicating that a Dialog
              n138 = Bundle By Name(cluster=T9 {"Multiplot XY Graph"=refnum, "Mouse Coordinates"={"Horizontal"=0, "Vertical"=0}, "Plot Index"=-1} ("Selected Plot Info"), "Multiplot XY Graph"=w338, "Mouse Coordinates"=w337) -> (w333:T9)
              n139 = Bundle("Selected Plot Info"=w333, "Dummy Scatter Plot Parameters\nindicating that a Dialog"=w335) -> (w332:T18)  [unwired: 1 in]
              n140 = Bundle By Name(cluster=T1 {"AlliGator Q Event"=enum."Phasor Graph:Parameter 2 vs Parameter 1 Scatter Plot", "Data"=variant} ("element"), "Data"=w332) -> (w339:T1)
              n141 = Build Array(w339) -> (w336:T1[])
            }
            frame "Parameter 2 vs Parameter 1 Scatter Plot (Selected Plots)" {
              w341 = T16 {"Parameter 2"=enum."Phasor g", "Parameter 1"=enum."Phasor g"}  # Dummy Scatter Plot Parameters indicating that a Dialog
              n142 = call "Selected Plots Mouse Coordinates Constant.vi"() -> ("Selected Plots Mouse Coordinates Equivalent"=w342:T4)
              n143 = Bundle By Name(cluster=T9 {"Multiplot XY Graph"=refnum, "Mouse Coordinates"={"Horizontal"=0, "Vertical"=0}, "Plot Index"=-1} ("Selected Plot Info"), "Multiplot XY Graph"=w347, "Mouse Coordinates"=w342) -> (w344:T9)
              n144 = Bundle("Selected Plot Info"=w344, "Dummy Scatter Plot Parameters\nindicating that a Dialog"=w341) -> (w343:T18)  [unwired: 1 in]
              n145 = Bundle By Name(cluster=T1 {"AlliGator Q Event"=enum."Phasor Graph:Parameter 2 vs Parameter 1 Scatter Plot", "Data"=variant} ("element"), "Data"=w343) -> (w348:T1)
              n146 = Build Array(w348) -> (w346:T1[])
            }
            frame "Parameter 2 vs Parameter 1 Scatter Plot (All Plots)" {
              w350 = T16 {"Parameter 2"=enum."Phasor g", "Parameter 1"=enum."Phasor g"}  # Dummy Scatter Plot Parameters indicating that a Dialog
              n147 = call "All Plots Mouse Coordinates Constant.vi"() -> ("Selected Plots Mouse Coordinates Equivalent"=w351:T4)
              n148 = Bundle By Name(cluster=T9 {"Multiplot XY Graph"=refnum, "Mouse Coordinates"={"Horizontal"=0, "Vertical"=0}, "Plot Index"=-1} ("Selected Plot Info"), "Multiplot XY Graph"=w356, "Mouse Coordinates"=w351) -> (w353:T9)
              n149 = Bundle("Selected Plot Info"=w353, "Dummy Scatter Plot Parameters\nindicating that a Dialog"=w350) -> (w352:T18)  [unwired: 1 in]
              n150 = Bundle By Name(cluster=T1 {"AlliGator Q Event"=enum."Phasor Graph:Parameter 2 vs Parameter 1 Scatter Plot", "Data"=variant} ("element"), "Data"=w352) -> (w357:T1)
              n151 = Build Array(w357) -> (w355:T1[])
            }
            frame "Compute Multiple Average Phasors (Selected Plots)" {
              n152 = Build Array(T1 {"AlliGator Q Event"=enum."Phasor Graph:Compute Multiple Average Phasors (Selected Plots)", "Data"=variant} ("element")) -> (w359:T1[])
            }
            frame "---------Export Add'l Phasor Plots Data (ASCII)------------" {
            }
            frame "Export Phasor Plot Data", "Export Single Phasor Plot Data" {
              n153 = Bundle By Name(cluster=T13 {"Mouse Click Event Data"={"Multiplot XY Graph"=refnum, "Mouse Coordinates"={"Horizontal"=0, "Vertical"=0}}, "Save as..."=FALSE} ("output cluster"), "Mouse Click Event Data.Multiplot XY Graph"=w368, "Mouse Click Event Data.Mouse Coordinates"=w367, "Save as..."=w366) -> (w362:T13)
              n154 = Bundle By Name(cluster=T1 {"AlliGator Q Event"=enum."Phasor Graph:Export Single Phasor Plot Data", "Data"=variant} ("element"), "Data"=w362) -> (w361:T1)
              n155 = Build Array(w361) -> (w365:T1[])
            }
            frame "Export Selected Phasor Plots Data" {
              w369 = FALSE  # Selected Plots
              n156 = Bundle By Name(cluster=T1 {"AlliGator Q Event"=enum."Phasor Graph:Export Selected Phasor Plots Data", "Data"=variant} ("element"), "Data"=w369) -> (w370:T1)
              n157 = Build Array(w370) -> (w372:T1[])
            }
            frame "Export All Phasor Plots Data" {
              w373 = TRUE  # All Plots
              n158 = Bundle By Name(cluster=T1 {"AlliGator Q Event"=enum."Phasor Graph:Export Selected Phasor Plots Data", "Data"=variant} ("element"), "Data"=w373) -> (w374:T1)
              n159 = Build Array(w374) -> (w376:T1[])
            }
            frame "------------------------------------" {
            }
            frame "Grid", "Show/Hide Grid" {
              n160 = call "XY Graph Show-Hide Grid Event.vi"("XYGraph Ref in"=w378) -> ("Message"=w377:string)  [unwired: 7 in, 3 out]
            }
            frame "Show/Hide Tool Panels", "Tool Panels" {
              n161 = call "XY Graph Show-Hide Tool Panels Event.vi"("XYGraph in"=w380) -> ("Message"=w379:string)  [unwired: 8 in, 2 out]
            }
          }
          n162 = case shown="True" w24 {
            tunnel: w22 -> [w25 w28]
            tunnel: [w25 w27] -> w18
            tunnel: T1 {"AlliGator Q Event"=enum."Phasor Plot:Update Phasor Plot Reference", "Data"=variant} ("element") -> [_ w26]
            frame False {
            }
            frame True {
              n163 = Build Array (concatenate)(w28, w26) -> (w27:T1[])
            }
          }
        }
        frame True {
          n164 = property class="XYGraph (strict)"(reference=w383) -> ("Label.Text"=w384:string)  [unwired: 1 in, 2 out]
          n165 = call "AlliGator Send Python Function Doc String to Notebook.vi"("Item Tag"=w382, "Target"=w384) -> ("Message"=w381:string)  [unwired: 8 in, 1 out]
        }
      }
    }
    frame Error {
    }
  }
  "AlliGator Actions" <- w6
  "Message" <- w1
  "Error Out" <- "Error In"
